vi "Loop_Timing_Fast_Loop.vi"(8 "error in":errorcluster, 10 "Outer Loop sample rate in":dbl=20.0, 11 "IMU_sample_rate in":i32=200) -> (0 "error out":errorcluster, 1 "Outer Loop Start":bool, 2 "30hz Start":bool, 3 "Hz":dbl format="%#_4g")   [LabVIEW 2014]
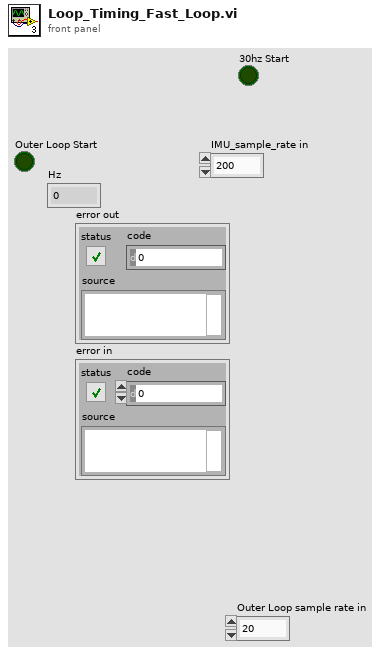
[diagram p1: front panel]
types:
  T1 = cluster{"Actual Hz":dbl, "Iteration Count":dbl, "Dt":dbl, "Average Hz":dbl}
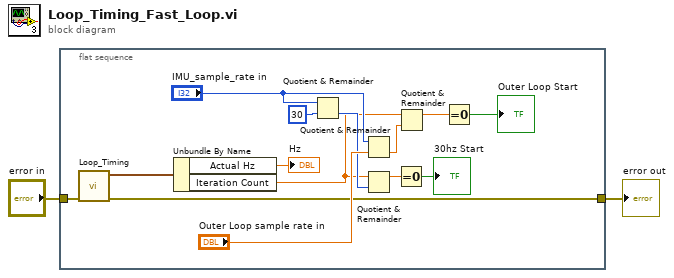
[diagram p0: block diagram]
diagram:
  n1 = flat-sequence {
    tunnel: "error in" -> [w5]
    tunnel: [w6] -> w1
    frame #0 {
      n2 = call "Loop_Timing.vi"("error in"=w5) -> ("error out"=w6:errorcluster, "Timing Block"=w7:T1)  [unwired: 9 in]
      n3 = Unbundle By Name(w7) -> ("Actual Hz"=→"Hz":dbl, "Iteration Count"=w3:dbl)
      n4 = Quotient & Remainder(x="IMU_sample_rate in", y=30) -> (floor(x/y)=w8:i32)  [unwired: 1 out]
      n5 = Quotient & Remainder(x="IMU_sample_rate in", y="Outer Loop sample rate in") -> (floor(x/y)=w14:dbl)  [unwired: 1 out]
      n6 = Quotient & Remainder(x=w3, y=w8) -> (x-y*floor(x/y)=w10:dbl)  [unwired: 1 out]
      n7 = Equal To 0?(x=w10) -> (x = 0?=→"30hz Start":bool)
      n8 = Quotient & Remainder(x=w3, y=w14) -> (x-y*floor(x/y)=w16:dbl)  [unwired: 1 out]
      n9 = Equal To 0?(x=w16) -> (x = 0?=→"Outer Loop Start":bool)
    }
  }
  "error out" <- w1
